vi "CAN Floats to Message.vi"(9 "Float_1":sgl, 10 "Float_0":sgl) -> (2 "CAN Message":u8[](array[numeric]))   [LabVIEW 2019]
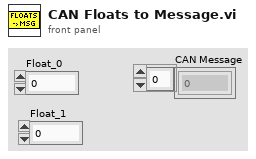
[diagram p1: front panel]
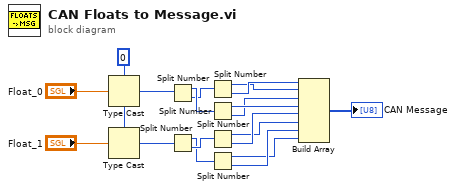
[diagram p0: block diagram]
diagram:
  w9 = u32 0 ("y")
  n1 = Type Cast(type=w9, x="Float_0") -> (*(type *) &x=w16:u32)
  n2 = Type Cast(type=w9, x="Float_1") -> (*(type *) &x=w6:u32)
  n3 = Split Number(x=w16) -> (hi(x)=w18:u16, lo(x)=w17:u16)
  n4 = Split Number(x=w6) -> (hi(x)=w7:u16, lo(x)=w8:u16)
  n5 = Split Number(x=w17) -> (hi(x)=w12:u8, lo(x)=w13:u8)
  n6 = Split Number(x=w18) -> (hi(x)=w15:u8, lo(x)=w14:u8)
  n7 = Split Number(x=w8) -> (hi(x)=w4:u8, lo(x)=w5:u8)
  n8 = Split Number(x=w7) -> (hi(x)=w2:u8, lo(x)=w3:u8)
  n9 = Build Array(w13, w12, w14, w15, w5, w4, w3, w2) -> (→"CAN Message":u8[])
